vi "pp2_NextState.vi"(6 "Actually run (passthrough if off)":bool=TRUE, 9 "New state countdown (ms)":i64 min=0, 10 "New State":T1=enum."2 (Load Trial)", 11 "State In":T2={"Curr  tr"=0, "Curr (ms)"=0, "Cum (ms)"=0, "Run loop diff"=0, "Tone countdown (ms)"=0, "Countdown (ms)"=0, "Curr State"=enum."0 NULL", "Prev State"=enum."1 Habituation", "Null"=FALSE, "Sw1"=FALSE, "Sw2"=FALSE, "Tone\nGate"=FALSE, "Stim"=FALSE, "Current DAQ DO Int"=0, "Current Loaded Trial"={"Trial Type Number"=1, "Trial Type"=enum."GO", "Trial Weight"=100, "Shock (mA)"=0.3, "Duration (ms)"=0.25, "Sound Type"=enum."04 FM Sweep", "Stim P1"=4000.0, "Stim P2"=0.0, "Stim P3"=0.0, "Stim P4"=2000.0}, "Next Trial (for display purposes)"={"Trial Type Number"=1, "Trial Type"=enum."GO", "Trial Weight"=100, "Shock (mA)"=0.3, "Duration (ms)"=0.25, "Sound Type"=enum."04 FM Sweep", "Stim P1"=4000.0, "Stim P2"=0.0, "Stim P3"=0.0, "Stim P4"=2000.0}, "Total trials memo"=0, "State start cum memo (ms)"=0, "Last dur jump time memo (ms)"=0, "Last dur shock time memo (ms)"=0, "Tone repeat memo"=0, "Webcam on"=FALSE, "Webcam recording"=FALSE} {"Current DAQ DO Int" format="%b"; "Next Trial (for display purposes)"."Shock (mA)" min=-1.0 max=5.0; "Next Trial (for display purposes)"."Trial Weight" step=1; "Next Trial (for display purposes)"."Duration (ms)" min=0.0 max=1.0; "Next Trial (for display purposes)"."Trial Type Number" min=1 step=1; "Current Loaded Trial"."Shock (mA)" min=-1.0 max=5.0; "Current Loaded Trial"."Trial Weight" step=1; "Current Loaded Trial"."Duration (ms)" min=0.0 max=1.0; "Current Loaded Trial"."Trial Type Number" min=1 step=1}) -> (3 "State Out":T2={"Curr  tr"=0, "Curr (ms)"=0, "Cum (ms)"=0, "Run loop diff"=0, "Tone countdown (ms)"=0, "Countdown (ms)"=0, "Curr State"=enum."0 NULL", "Prev State"=enum."1 Habituation", "Null"=FALSE, "Sw1"=FALSE, "Sw2"=FALSE, "Tone\nGate"=FALSE, "Stim"=FALSE, "Current DAQ DO Int"=0, "Current Loaded Trial"={"Trial Type Number"=1, "Trial Type"=enum."GO", "Trial Weight"=100, "Shock (mA)"=0.3, "Duration (ms)"=0.25, "Sound Type"=enum."04 FM Sweep", "Stim P1"=4000.0, "Stim P2"=0.0, "Stim P3"=0.0, "Stim P4"=2000.0}, "Next Trial (for display purposes)"={"Trial Type Number"=1, "Trial Type"=enum."GO", "Trial Weight"=100, "Shock (mA)"=0.3, "Duration (ms)"=0.25, "Sound Type"=enum."04 FM Sweep", "Stim P1"=4000.0, "Stim P2"=0.0, "Stim P3"=0.0, "Stim P4"=2000.0}, "Total trials memo"=0, "State start cum memo (ms)"=0, "Last dur jump time memo (ms)"=0, "Last dur shock time memo (ms)"=0, "Tone repeat memo"=0, "Webcam on"=FALSE, "Webcam recording"=FALSE} {"Current DAQ DO Int" format="%b"; "Next Trial (for display purposes)"."Shock (mA)" min=-1.0 max=5.0; "Next Trial (for display purposes)"."Trial Weight" step=1; "Next Trial (for display purposes)"."Duration (ms)" min=0.0 max=1.0; "Next Trial (for display purposes)"."Trial Type Number" min=1 step=1; "Current Loaded Trial"."Shock (mA)" min=-1.0 max=5.0; "Current Loaded Trial"."Trial Weight" step=1; "Current Loaded Trial"."Duration (ms)" min=0.0 max=1.0; "Current Loaded Trial"."Trial Type Number" min=1 step=1})   [LabVIEW 2013]
uses:
  pp2_CTL_StateInfo.ctl
  pp2_CTL_State.ctl
  pp2_Trial.ctl
  pp2_CTL_TrialType.ctl
  labolabo2/waveforms/WFTypes.ctl
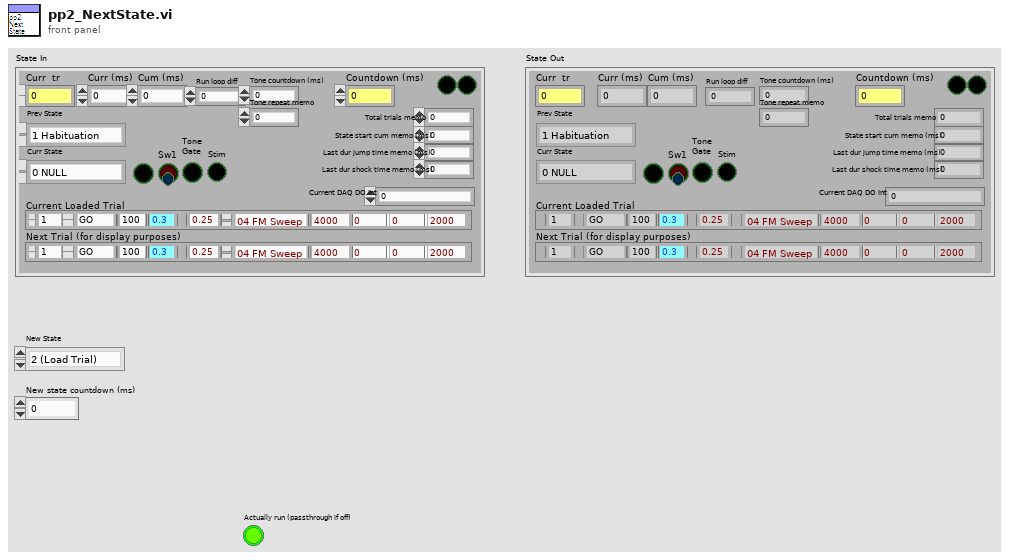
[diagram p1: front panel]
types:
  T1 = typedef "pp2_CTL_State.ctl" = enum8{"0 NULL", "1 Habituation", "2 (Load Trial)", "3 Stay Period", "4 (Load Audio)", "5 GO Trial", "6 GO Jumped", "7 GO Timeout", "8 NOGO Trial", "9 NOGO Jumped", "10 NOGO Timeout", "11 TEST Trial", "12 TEST Jumped", "13 TEST Timeout", "14 Intertrial Interval"}
  T2 = typedef "pp2_CTL_StateInfo.ctl" = cluster{"Curr  tr":u16, "Curr (ms)":i64, "Cum (ms)":i64, "Run loop diff":i64, "Tone countdown (ms)":i64, "Countdown (ms)":i64, "Curr State":T1, "Prev State":T1, "Null":bool, "Sw1":bool, "Sw2":bool, "Tone\nGate":bool, "Stim":bool, "Current DAQ DO Int":u16, "Current Loaded Trial":T3, "Next Trial (for display purposes)":T3, "Total trials memo":i64, "State start cum memo (ms)":i64, "Last dur jump time memo (ms)":i64, "Last dur shock time memo (ms)":i64, "Tone repeat memo":i64, "Webcam on":bool, "Webcam recording":bool}
  T3 = typedef "pp2_Trial.ctl" = cluster{"Trial Type Number":u8, "Trial Type":T4, "Trial Weight":u32, "Shock (mA)":dbl, "Duration (ms)":dbl, "Sound Type":T5, "Stim P1":dbl, "Stim P2":dbl, "Stim P3":dbl, "Stim P4":dbl}
  T4 = typedef "pp2_CTL_TrialType.ctl" = enum16{"OFF", "GO", "NOGO", "TEST"}
  T5 = typedef "WFTypes.ctl" = enum16{"00 NULL", "01 DC", "02 Noise", "03 Pure Tone", "04 FM Sweep"}
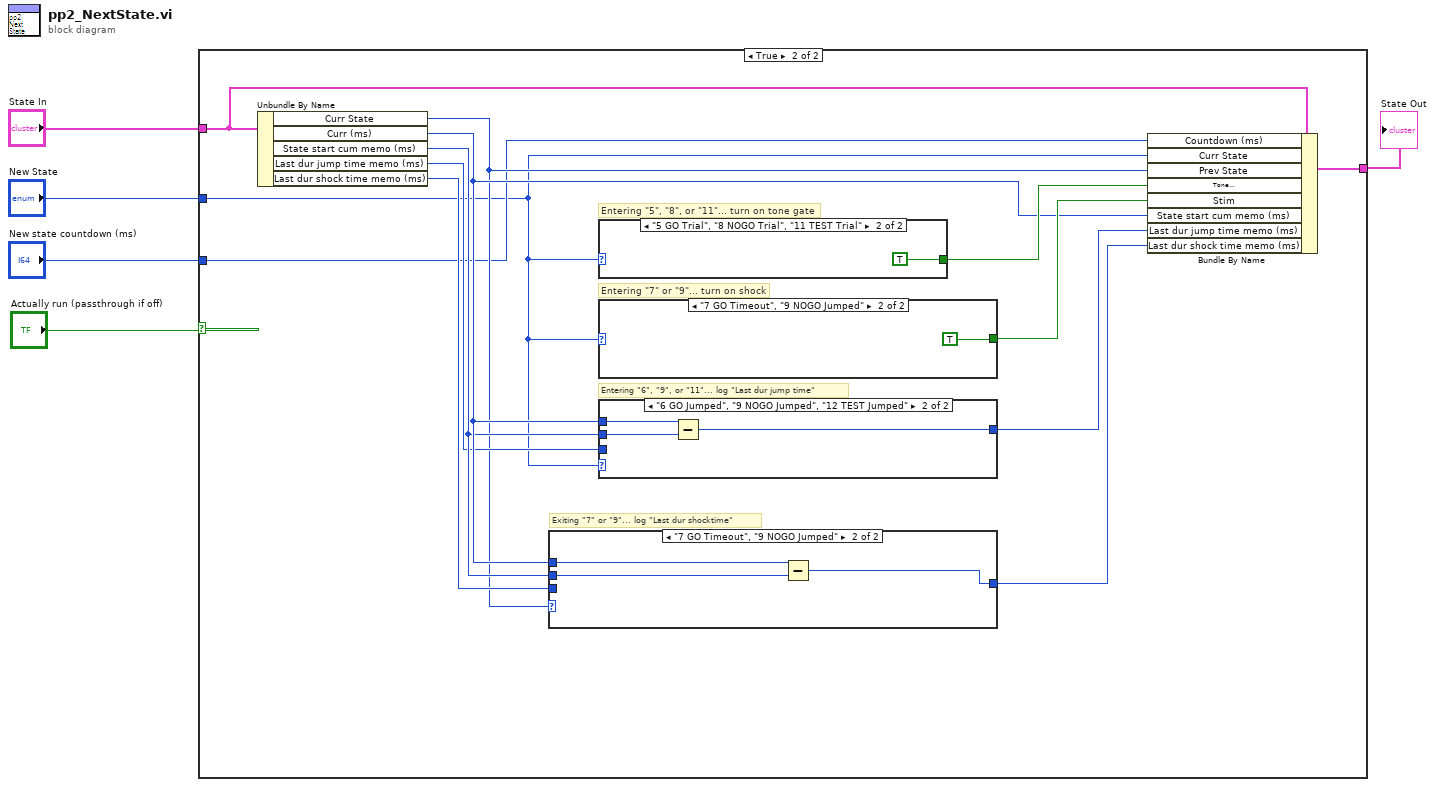
[diagram p0: block diagram]
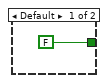
[diagram p5: hidden frame]
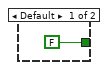
[diagram p6: hidden frame]
diagram:
  n1 = case shown="True" "Actually run (passthrough if off)" {
    tunnel: [w6 w19] -> w5
    tunnel: "New state countdown (ms)" -> [_ w8]
    tunnel: "State In" -> [w6 w18]
    tunnel: "New State" -> [_ w7]
    frame False {
    }
    frame True {
      # "Entering \"7\" or \"9\"... turn on shock"
      # "Entering \"6\", \"9\", or \"11\"... log \"Last dur jump time\""
      # "Entering \"5\", \"8\", or \"11\"... turn on tone gate"
      # "Exiting \"7\" or \"9\"... log \"Last dur shocktime\""
      n2 = Unbundle By Name(w18) -> ("Curr State"=w9:T1, "Curr (ms)"=w14:i64, "State start cum memo (ms)"=w13:i64, "Last dur jump time memo (ms)"=w12:i64, "Last dur shock time memo (ms)"=w10:i64)
      n3 = case shown="\"7 GO Timeout\", \"9 NOGO Jumped\"" w9 {
        tunnel: w13 -> [_ w22]
        tunnel: w14 -> [_ w23]
        tunnel: w10 -> [w20 _]
        tunnel: [w20 w21] -> w11
        frame Default {
        }
        frame "7 GO Timeout", "9 NOGO Jumped" {
          n4 = Subtract(x=w23, y=w22) -> (x-y=w21:i64)
        }
      }
      n5 = case shown="\"5 GO Trial\", \"8 NOGO Trial\", \"11 TEST Trial\"" w7 {
        tunnel: [FALSE TRUE] -> w17
        frame Default {
        }
        frame "5 GO Trial", "8 NOGO Trial", "11 TEST Trial" {
        }
      }
      n6 = case shown="\"7 GO Timeout\", \"9 NOGO Jumped\"" w7 {
        tunnel: [FALSE TRUE] -> w16
        frame Default {
        }
        frame "7 GO Timeout", "9 NOGO Jumped" {
        }
      }
      n7 = case shown="\"6 GO Jumped\", \"9 NOGO Jumped\", \"12 TEST Jumped\"" w7 {
        tunnel: w13 -> [_ w26]
        tunnel: w14 -> [_ w27]
        tunnel: w12 -> [w24 _]
        tunnel: [w24 w25] -> w15
        frame Default {
        }
        frame "6 GO Jumped", "9 NOGO Jumped", "12 TEST Jumped" {
          n8 = Subtract(x=w27, y=w26) -> (x-y=w25:i64)
        }
      }
      n9 = Bundle By Name(cluster=w18, "Countdown (ms)"=w8, "Curr State"=w7, "Prev State"=w9, "Tone\nGate"=w17, "Stim"=w16, "State start cum memo (ms)"=w14, "Last dur jump time memo (ms)"=w15, "Last dur shock time memo (ms)"=w11) -> (w19:T2)
    }
  }
  "State Out" <- w5
